vi "poll_ARM.vi"(10 "Seconds to wait\nbefore reading ARM":u32=6, 11 "ARM COM":refnum<visa-resource-name>="COM4") -> (1 "ARM Reply":string="00000\t07/02/2019 17:17:56\t11.97\t0.630427\t0.000039\t-1.173338\t0.000042\t-0.923238\t0.000014\t0.000229\t0.000263\t\r\r\ný")   [LabVIEW 2022 SP3]
uses:
  <vilib>/Instr/_visa.llb/VISA Configure Serial Port (Instr).vi
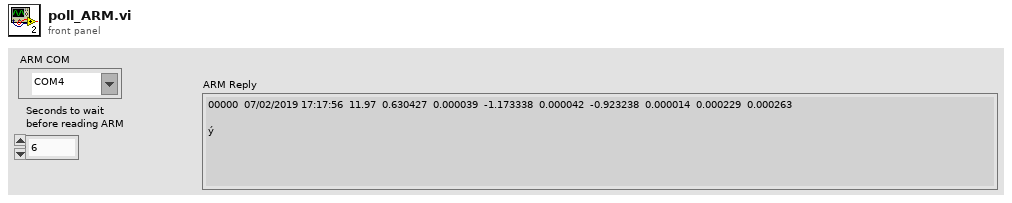
[diagram p1: front panel]
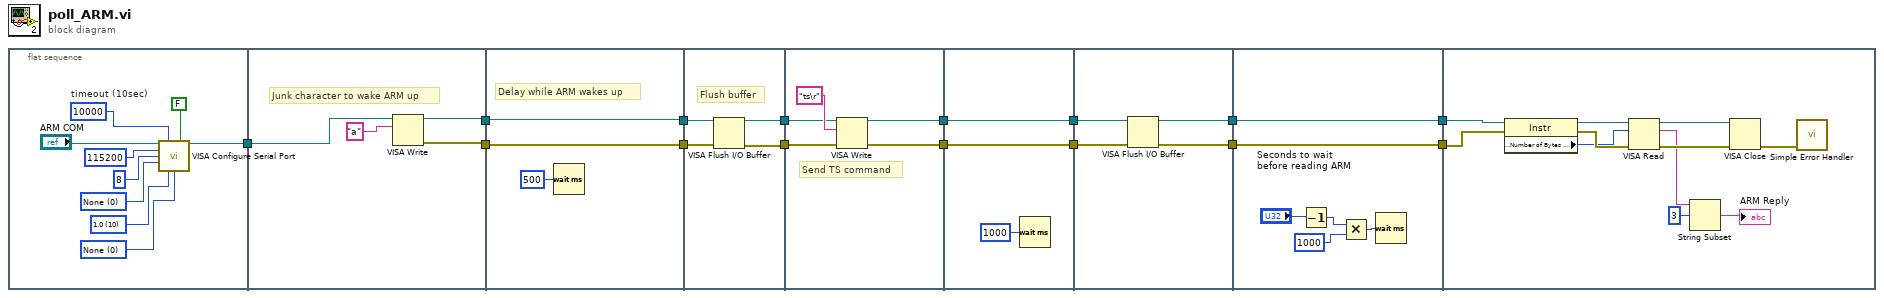
[diagram p0: block diagram]
diagram:
  n1 = flat-sequence {
    tunnel: [w16] -> w7
    tunnel: [w27] -> w15
    tunnel: [w26] -> w14
    tunnel: w7 -> [w25]
    tunnel: [w31] -> w13
    tunnel: w15 -> [w31]
    tunnel: [w30] -> w12
    tunnel: w14 -> [w30]
    tunnel: w13 -> [w35]
    tunnel: [w33] -> w11
    tunnel: w12 -> [w34]
    tunnel: [w32] -> w10
    tunnel: w11 -> [w39]
    tunnel: w10 -> [w38]
    tunnel: [w36] -> w6
    tunnel: [w37] -> w5
    tunnel: w6 -> [w43]
    tunnel: [w43] -> w4
    tunnel: w5 -> [w42]
    tunnel: [w42] -> w2
    tunnel: w4 -> [w46]
    tunnel: [w45] -> w3
    tunnel: w2 -> [w47]
    tunnel: [w44] -> w1
    tunnel: [w53] -> w9
    tunnel: w3 -> [w52]
    tunnel: [w52] -> w8
    tunnel: w1 -> [w53]
    tunnel: w9 -> [w61]
    tunnel: w8 -> [w60]
    frame #0 {
      w22 = u16 0 items=["None"=0, "XON/XOFF"=1, "RTS/CTS"=2, "DTR/DSR"=4] ("Flow Control")
      w21 = u16 10 items=["1.0"=10, "1.5"=15, "2.0"=20] ("Stop Bits")
      w18 = u16 0 items=["None", "Odd", "Even", "Mark", "Space"] ("Parity")
      w24 = u32 10000  # timeout (10sec)
      n2 = call-poly "VISA Configure Serial Port"("VISA resource name"="ARM COM", "timeout (10sec)"=w24, "Enable Termination\nChar (T)"=FALSE ("Enable Termination Char (T)"), "baud rate (9600)"=u32 115200 ("Baud Rate"), "data bits (8)"=u16 8 ("Data Bits"), "parity (0:none)"=w18, "stop bits (10: 1 bit)"=w21, "flow control (0:none)"=w22) -> ("VISA resource name out"=w16:refnum<visa-resource-name>)  [unwired: 1 in, 6 out]
    }
    frame #1 {
      # "Junk character to wake ARM up"
      n3 = VISA Write(VISA resource name=w25, write buffer="a") -> (VISA resource name out=w27:refnum<visa-resource-name>, error out=w26:errorcluster)  [unwired: 1 in, 1 out]
    }
    frame #2 {
      # "Delay while ARM wakes up"
      n4 = Wait (ms)(milliseconds to wait=u32 500) -> ()  [unwired: 1 out]
    }
    frame #3 {
      # "Flush buffer"
      n5 = VISA Flush I/O Buffer(VISA resource name=w35, error in (no error)=w34) -> (VISA resource name out=w33:refnum<visa-resource-name>, error out=w32:errorcluster)  [unwired: 1 in]
    }
    frame #4 {
      # "Send TS command"
      n6 = VISA Write(VISA resource name=w39, write buffer="ts\r", error in (no error)=w38) -> (VISA resource name out=w37:refnum<visa-resource-name>, error out=w36:errorcluster)  [unwired: 1 out]
    }
    frame #5 {
      n7 = Wait (ms)(milliseconds to wait=u32 1000) -> ()  [unwired: 1 out]
    }
    frame #6 {
      n8 = VISA Flush I/O Buffer(VISA resource name=w47, error in (no error)=w46) -> (VISA resource name out=w44:refnum<visa-resource-name>, error out=w45:errorcluster)  [unwired: 1 in]
    }
    frame #7 {
      n9 = Decrement(x="Seconds to wait\nbefore reading ARM") -> (x-1=w48:u32)
      n10 = Multiply(x=w48, y=u32 1000) -> (x*y=w50:u32)
      n11 = Wait (ms)(milliseconds to wait=w50) -> ()  [unwired: 1 out]
    }
    frame #8 {
      n12 = property class="Instr"(reference=w61, error in=w60) -> (reference out=w64:refnum<visa-resource-name>, error out=w63:errorcluster, "Serial Settings:Number of Bytes at Serial Port"=w62:u32)
      n13 = VISA Read(VISA resource name=w64, byte count=w62, error in (no error)=w63) -> (VISA resource name out=w59:refnum<visa-resource-name>, read buffer=w56:string, error out=w58:errorcluster)  [unwired: 1 out]
      n14 = String Subset(string=w56, offset (0)=3) -> (substring=→"ARM Reply":string)  [unwired: 1 in]
      n15 = VISA Close(VISA resource name=w59, error in (no error)=w58) -> (error out=w57:errorcluster)
      n16 = call <vilib>:"Simple Error Handler.vi"("error in (no error)"=w57) -> ()  [unwired: 1 in, 8 out]
    }
  }
